vi "_script_fix_exclude event case ref check.vi"   [LabVIEW 2014]
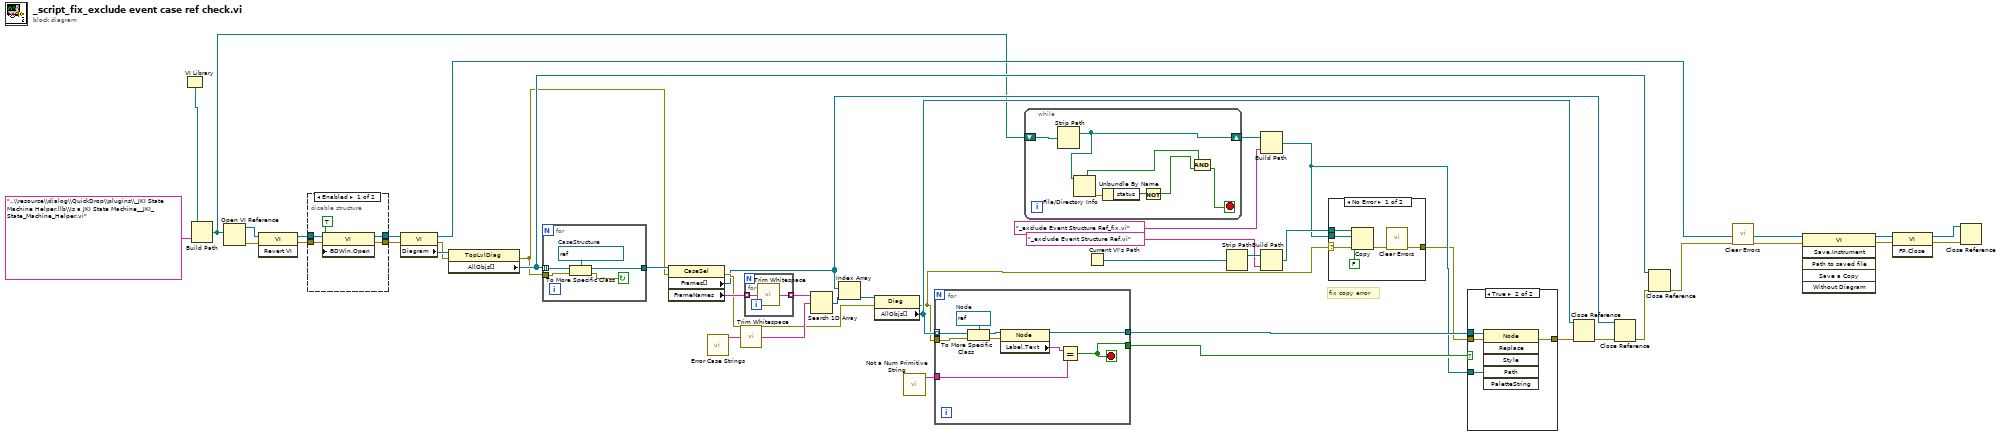
[diagram p0: block diagram]
diagram:
  # "fix copy error"
  n1 = VI Library() -> (path=w43:path)
  n2 = Build Path(base path=w43, name or relative path="..\\resource\\dialog\\QuickDrop\\plugins\\_JKI State Machine Helper.llb\\Is a JKI State Machine__JKI_State_Machine_Helper.vi") -> (appended path=w14:path)
  n3 = Open VI Reference(vi path=w14) -> (vi reference=w44:refnum<vi>, error out=w45:errorcluster)  [unwired: 5 in]
  n4 = invoke class="VI" method="Revert VI"(reference=w44, error in=w45) -> (reference out=w41:refnum<vi>, error out=w40:errorcluster)  [unwired: 1 in, 1 out]
  n5 = disable-structure shown="Enabled" {
    disable-tunnel: w41 -> [w50 w52]
    disable-tunnel: w40 -> [w49 w51]
    disable-tunnel: [w48 w52] -> w39
    disable-tunnel: [w47 w51] -> w38
    frame Enabled {
      n6 = property class="VI"(reference=w50, error in=w49, "BDWin.Open"=TRUE ("Block Diagram Window:Open")) -> (reference out=w48:refnum<vi>, error out=w47:errorcluster)
    }
    frame Disabled {
    }
  }
  n7 = property class="VI"(reference=w39, error in=w38) -> (reference out=w34:refnum<vi>, error out=w36:errorcluster, "Diagram"=w37:refnum<vi>)
  n8 = property class="TopLvlDiag"(reference=w37, error in=w36) -> (error out=w26:errorcluster, "AllObjs[]"=w32:refnum<vi>[])  [unwired: 1 out]
  n9 = for {
    tunnel: w32 -> [w57] mode=indexing
    tunnel: [w53] -> w35
    tunnel: w26 -> [w55]
    stop <- w54 continue-if-true
    w56 = refnum<vi> refnum  # CaseStructure
    n10 = To More Specific Class(target class=w56, reference=w57, error in=w55) -> (specific class reference=w53:refnum<vi>, error out=w54:errorcluster)
  }
  n11 = property class="CaseSel"(reference=w35, error in=w26) -> (error out=w25:errorcluster, "Frames[]"=w19:refnum<vi>[], "FrameNames"=w31:string[])  [unwired: 1 out]
  n12 = call "Error Case Strings.vi"() -> ("No Error"=w7:string)  [unwired: 10 in, 1 out]
  n13 = call <vilib>:"Trim Whitespace.vi"("string"=w7) -> ("trimmed string"=w29:string)  [unwired: 1 in]
  n14 = for {
    tunnel: w31 -> [w59] mode=indexing
    tunnel: [w58] -> w30 mode=indexing
    n15 = call <vilib>:"Trim Whitespace.vi"("string"=w59) -> ("trimmed string"=w58:string)  [unwired: 1 in]
  }
  n16 = Search 1D Array(1D array=w30, element=w29) -> (index of element=w28:i32)  [unwired: 1 in]
  n17 = Index Array(array=w19, index=w28) -> (element=w27:refnum<vi>)
  n18 = property class="Diag"(reference=w27, error in=w25) -> (error out=w12:errorcluster, "AllObjs[]"=w20:refnum<vi>[])  [unwired: 1 out]
  n19 = call "Not a Num Primitive String.vi"() -> ("Error"=w6:string)  [unwired: 10 in]
  n20 = for {
    tunnel: w20 -> [w68] mode=indexing
    tunnel: w12 -> [w66]
    tunnel: [w62] -> w24
    tunnel: [w61] -> w11
    tunnel: w6 -> [w60]
    stop <- w61 stop-if-true
    w67 = refnum<vi> refnum  # Node
    n21 = To More Specific Class(target class=w67, reference=w68, error in=w66) -> (specific class reference=w65:refnum<vi>, error out=w64:errorcluster)
    n22 = property class="Node"(reference=w65, error in=w64) -> (reference out=w62:refnum<vi>, "Label.Text"=w63:string)  [unwired: 1 out]
    n23 = Equal?(x=w63, y=w60) -> (x = y?=w61:bool)
  }
  n24 = while {
    shift-right: [w71] -> w15
    shift-left: w14 -> [w75]
    stop <- w74 stop-if-true
    n25 = Strip Path(path=w75) -> (stripped path=w71:path)  [unwired: 1 out]
    n26 = File/Directory Info(path=w71) -> (directory=w70:bool, error out=w73:errorcluster)  [unwired: 1 in, 5 out]
    n27 = Unbundle By Name(w73) -> ("status"=w72:bool)
    n28 = Not(x=w72) -> (.not. x?=w69:bool)
    n29 = And(x=w70, y=w69) -> (x .and. y?=w74:bool)
  }
  n30 = Current VI's Path() -> (path=w23:path)
  n31 = Strip Path(path=w23) -> (stripped path=w22:path)  [unwired: 1 out]
  n32 = Build Path(base path=w15, name or relative path="_exclude Event Structure Ref_fix.vi") -> (appended path=w10:path)
  n33 = Build Path(base path=w22, name or relative path="_exclude Event Structure Ref.vi") -> (appended path=w16:path)
  n34 = case shown="No Error" w12 {
    selector: w12 -> [w79 w82]
    tunnel: w16 -> [w81 _]
    tunnel: w10 -> [w77 _]
    tunnel: [w76 w82] -> w8
    frame No Error {
      n35 = Copy(8:w79, 9:FALSE ("overwrite (F)"), 10:w77, 11:w81) -> (0:w78:errorcluster)  [unwired: 1 in, 2 out]
      n36 = call <vilib>:"Clear Errors.vi"("error in (no error)"=w78) -> ("error out"=w76:errorcluster)  [unwired: 5 in, 1 out]
    }
    frame Error {
    }
  }
  n37 = case shown="True" w11 {
    tunnel: w24 -> [_ w87]
    tunnel: [w83 w86] -> w21
    tunnel: w8 -> [w83 w85]
    tunnel: w10 -> [_ w84]
    frame False {
    }
    frame True {
      n38 = invoke class="Node" method="Replace"(reference=w87, error in=w85, "Path"=w84) -> (error out=w86:errorcluster)  [unwired: 3 in, 5 out]
    }
  }
  n39 = Close Reference(reference=w20, error in (no error)=w21) -> (error out=w18:errorcluster)
  n40 = Close Reference(reference=w19, error in (no error)=w18) -> (error out=w17:errorcluster)
  n41 = Close Reference(reference=w32, error in (no error)=w17) -> (error out=w33:errorcluster)
  n42 = call <vilib>:"Clear Errors.vi"("error in (no error)"=w33) -> ("error out"=w1:errorcluster)  [unwired: 5 in, 1 out]
  n43 = invoke class="VI" method="Save.Instrument"(reference=w34, error in=w1) -> (reference out=w4:refnum<vi>, error out=w5:errorcluster)  [unwired: 4 in, 4 out]
  n44 = invoke class="VI" method="FP.Close"(reference=w4, error in=w5) -> (reference out=w2:refnum<vi>, error out=w3:errorcluster)  [unwired: 1 in, 1 out]
  n45 = Close Reference(reference=w2, error in (no error)=w3) -> ()  [unwired: 1 out]
